vi "Wave gage cal.vi"(0 "refnum in":refnum<k5>, 11 "Uncalibrated index":u32, 12 "Reference Index":u32) -> ()   [LabVIEW 2010]
uses:
  global scale array.vi
  DataServer/command.ctl
  DataServer/command cluster.ctl
  DAC apps/support/method.ctl
panel:
  in  "method":T1={"sampling interval"=0.1, "samples to average"=1, "data interval"=0.0, "stream data"=FALSE, "file path"=refnum, "command"={"command"=enum."Idle", "start time (ms)"=0, "Channel Indices"=[], "Scans per Sample"=1}} {"command"."Scans per Sample" min=1; "data interval" format="%.2f"; "samples to average" min=1 step=1; "sampling interval" format="%.2f"}
  # "s"
  # "s"
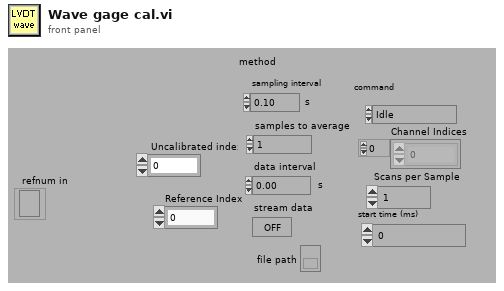
[diagram p1: front panel]
types:
  T1 = typedef "method.ctl" = cluster{"sampling interval":sgl, "samples to average":u32, "data interval":sgl, "stream data":bool, "file path":refnum<file>, "command":T2}
  T2 = typedef "command cluster.ctl" = cluster{"command":T3, "start time (ms)":u32, "Channel Indices":i32[], "Scans per Sample":i32}
  T3 = typedef "command.ctl" = enum16{"Idle", "Send Data", "Send 1 Scan", "Logoff"}
  T4 = enum16{"Volts", "Polynomial", "Correspondence Table", "pH", "Dissolved Oxygen", "Quadratic"}
  T5 = typedef "calib array.ctl" = T6[]
  T6 = typedef "conversion.ctl" = cluster{"conversion matrix":sgl[][], "units":string, "name":string, "scale type":T7, "offset (volts)":dbl, "second channel":i8, "correspondence table":T8, "offset (physical units)":dbl, "pH scale":T9, "D.O.":T10}
  T7 = typedef "scale type.ctl" = enum16{"Volts", "Polynomial", "Correspondence Table", "pH", "Dissolved Oxygen", "Quadratic"}
  T8 = typedef "correspondence table.ctl" = cluster{"physical units":dbl, "volts":dbl}[]
  T9 = typedef "pH scale.ctl" = cluster{"Buffers":cluster{"Buffer":dbl, "Calibrated":bool, "V/T":dbl}[], "Temperature":dbl}
  T10 = typedef "DO scale.ctl" = cluster{"Temperature":dbl, "K":dbl, "barometric pressure":dbl}
  T11 = enum16{"Volts", "Polynomial", "Correspondence Table", "pH", "Dissolved Oxygen"}
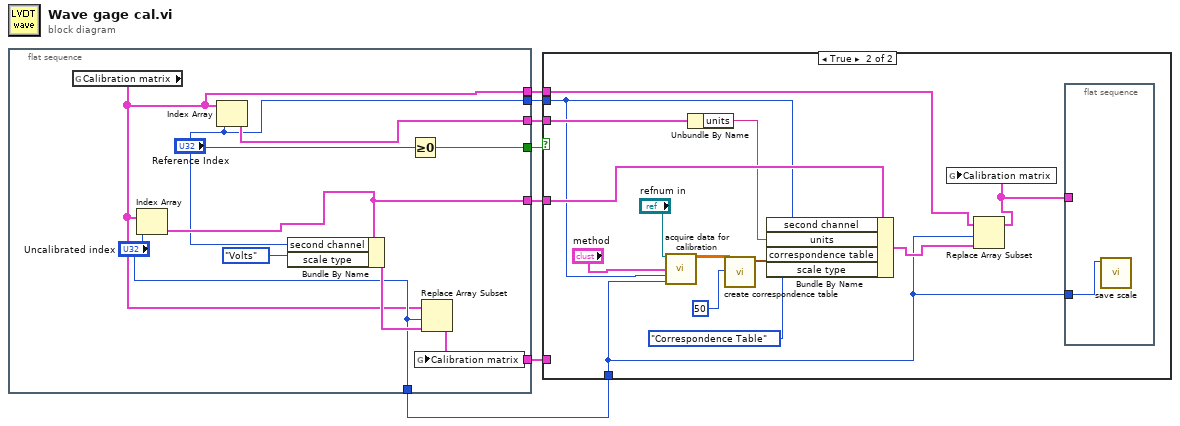
[diagram p0: block diagram]
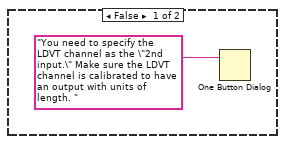
[diagram p2: hidden frame]
diagram:
  n1 = flat-sequence {
    tunnel: [w14] -> w7
    tunnel: [w13] -> w6
    tunnel: [w12] -> w5
    tunnel: ["Reference Index"] -> w4
    tunnel: ["Uncalibrated index"] -> w1
    tunnel: [w9] -> w3
    tunnel: [w8] -> w2
    frame #0 {
      n2 = global read "global scale array.vi" "Calibration matrix"() -> (w8:T5)
      n3 = Index Array(array=w8, index="Uncalibrated index") -> (element=w12:T6)
      n4 = Index Array(array=w8, index="Reference Index") -> (element=w13:T6)
      n5 = Bundle By Name(cluster=w12, "second channel"="Reference Index", "scale type"=T4."Volts") -> (w15:T6)
      n6 = Greater Or Equal To 0?(x="Reference Index") -> (x >= 0?=w14:bool)
      n7 = Replace Array Subset(array=w8, new element=w15, index="Uncalibrated index") -> (w9:T5)
      n8 = global write "global scale array.vi" "Calibration matrix"(w9) -> ()
    }
  }
  n9 = case shown="True" w7 {
    tunnel: w5 -> [_ w30]
    tunnel: w6 -> [_ w26]
    tunnel: w4 -> [_ w20]
    tunnel: w3 -> [_ _]
    tunnel: w2 -> [_ w21]
    tunnel: w1 -> [_ w18]
    frame False {
      n10 = One Button Dialog(message="You need to specify the LDVT channel as the \"2nd input.\" Make sure the LDVT channel is calibrated to have an output with units of length. ") -> ()  [unwired: 1 in, 1 out]
    }
    frame True {
      n11 = call "acquire data for calibration.vi"("Connection ID"="refnum in", "method"="method", "Reference Index"=w20, "Uncalibrated index"=w18) -> ("data array"=w28:sgl[][])  [unwired: 9 in, 2 out]
      n12 = Unbundle By Name(w26) -> ("units"=w25:string)
      n13 = call "create correspondence table.vi"("pieces"=50, "data array"=w28) -> ("correspondence table"=w29:T8)  [unwired: 8 in, 1 out]
      n14 = Bundle By Name(cluster=w30, "second channel"=w20, "units"=w25, "correspondence table"=w29, "scale type"=T11."Correspondence Table" ("Bundle Element")) -> (w22:T6)
      n15 = Replace Array Subset(array=w21, new element=w22, index=w18) -> (w19:T5)
      n16 = global write "global scale array.vi" "Calibration matrix"(w19) -> ()
      n17 = flat-sequence {
        tunnel: w19 -> [_]
        tunnel: w18 -> [w32]
        frame #0 {
          n18 = call "save scale.vi"("Index"=w32) -> ()  [unwired: 6 in, 1 out]
        }
      }
    }
  }
